vi "DAQNaviGet_DI_PortCount.vi"(8 "error in (no error)":errorcluster, 11 "task in":i32) -> (0 "error out":errorcluster, 2 "port count":i32, 3 "task out":i32)   [LabVIEW 2020]
uses:
  DAQNavi_LV.dll
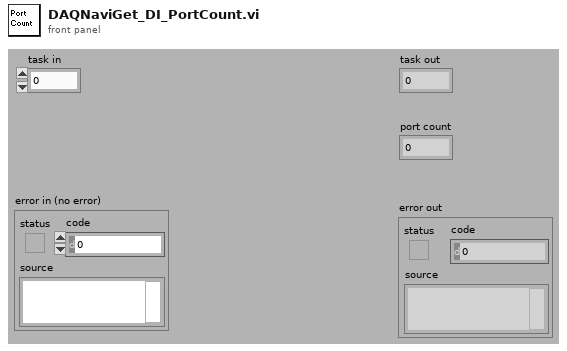
[diagram p1: front panel]
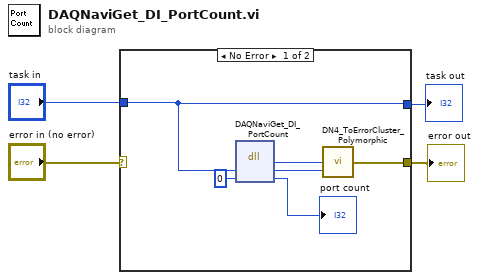
[diagram p0: block diagram]
diagram:
  n1 = case shown="No Error" "error in (no error)" {
    selector: "error in (no error)" -> [_ w11]
    tunnel: "task in" -> [w6 w12]
    tunnel: [w7 w11] -> w2
    tunnel: [w6 w12] -> w1
    frame No Error {
      n2 = dll-call lib="DAQNavi_LV.dll" fn="DAQNaviGet_DI_PortCount"("taskID"=w6, "portCount"=0 ("channelCount")) -> ("return type"=w8:i32, "taskID"=w5:i32, "portCount"=→"port count":i32)  [unwired: 3 in, 2 out]
      n3 = call "DN4_ToErrorCluster_Polymorphic.vi"("task id"=w5, "error code"=w8) -> ("error out"=w7:errorcluster)  [unwired: 3 out]
    }
    frame Error {
    }
  }
  "task out" <- w1
  "error out" <- w2
